vi "PFI-28000-System_Get Cards.vi"(8 "error in (no error)":errorcluster, 11 "PFI-28000-System in":refnum<class "PFI-28000-System.lvclass">) -> (0 "error out":errorcluster, 2 "Cards":refnum<class "PFI-28000-Card.lvclass">[](array[class]), 3 "PFI-28000-System out":refnum<class "PFI-28000-System.lvclass">)   [LabVIEW 2017, in "PFI-28000-System.lvclass"]
uses:
  PFI-28000-System.lvclass
  Card/PFI-28000-Card.lvclass
  PFI-28000-System.lvclass/PFI-28000-System.ctl
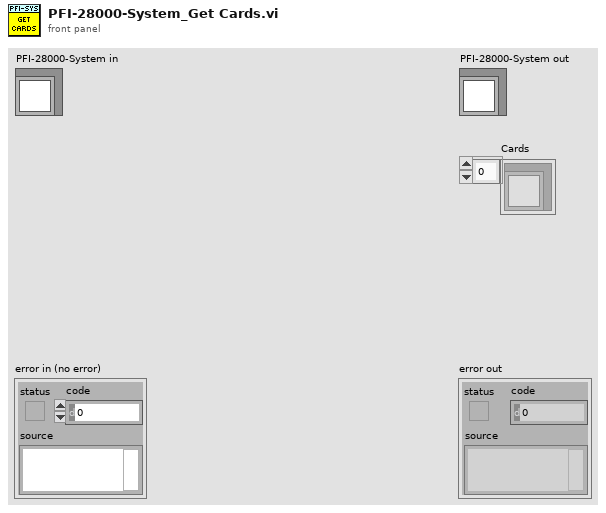
[diagram p1: front panel]
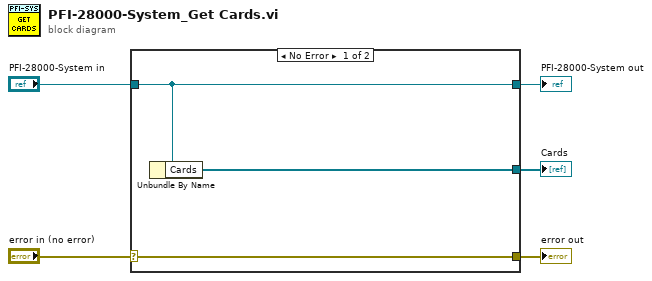
[diagram p0: block diagram]
diagram:
  n1 = case shown="No Error" "error in (no error)" {
    selector: "error in (no error)" -> [w8 w9]
    tunnel: [w8 w9] -> w4
    tunnel: [w7 w10] -> w2
    tunnel: "PFI-28000-System in" -> [w7 w10]
    tunnel: [w6 _] -> w1
    frame No Error {
      n2 = Unbundle By Name(w7) -> ("Cards"=w6:refnum<class "PFI-28000-Card.lvclass">[])
    }
    frame Error {
    }
  }
  "error out" <- w4
  "PFI-28000-System out" <- w2
  "Cards" <- w1
